vi "show_tag_status.vi"(11 "file path (dialog if empty)":path=path "c:/RFID/status.csv") -> (2 "Output":T2, 3 "train_passes_text":string)   [LabVIEW 2015]
uses:
  <vilib>/Utility/file.llb/Read Delimited Spreadsheet (string).vi
panel:
  out "all rows":string[][](array[string])
  in  "Cluster":T1
  out "subarray":string[](array[string])
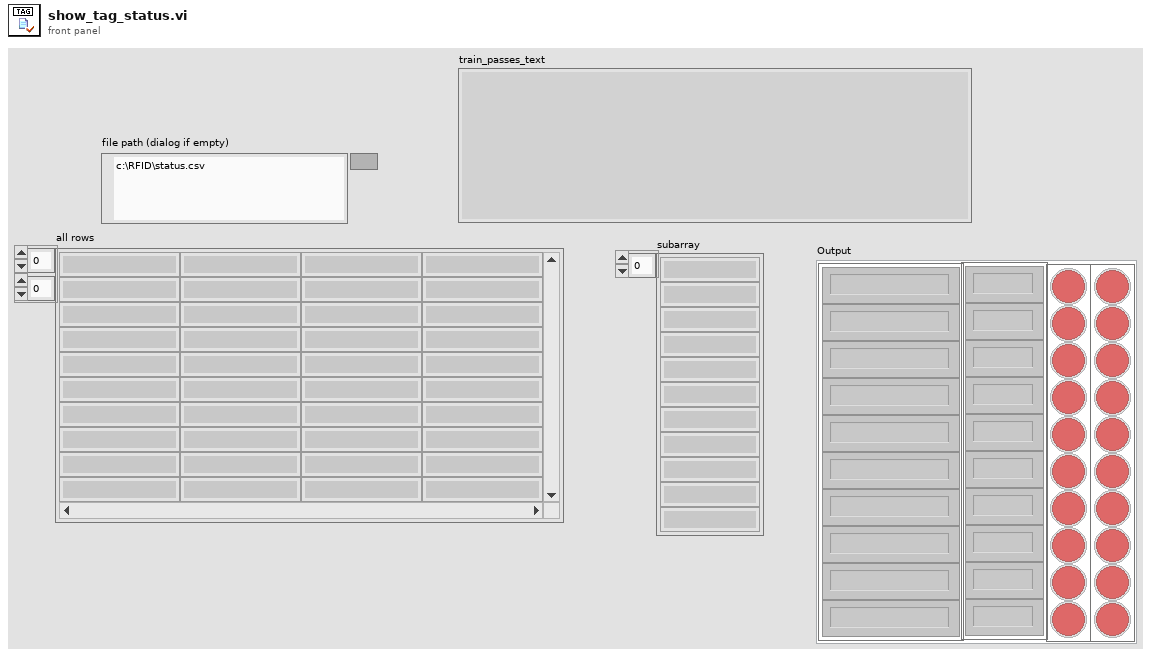
[diagram p1: front panel]
types:
  T1 = cluster{"Array 3":bool[], "Array 1":string[], "Array 2":string[], "Array 4":bool[]}
  T2 = cluster{"Array 3":bool[], "Array 4":string[], "Array 6":string[], "Array 5":bool[]}
  T3 = enum16{"open", "replace", "create", "open or create", "replace or create", "replace or create with confirmation"}
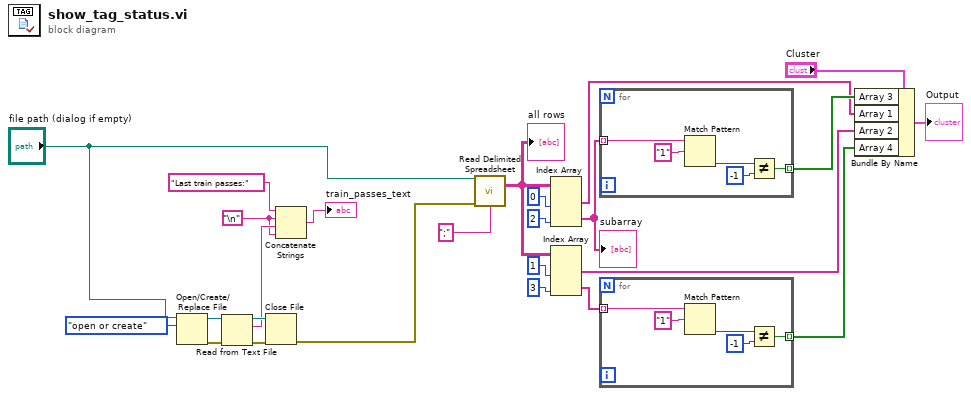
[diagram p0: block diagram]
diagram:
  w3 = "\n"
  n1 = Open/Create/Replace File(file path (use dialog)="file path (dialog if empty)", operation (0:open)=T3."open or create") -> (refnum out=w8:refnum<file>, error out=w10:errorcluster)  [unwired: 4 in, 1 out]
  n2 = Read from Text File(file (use dialog)=w8, error in=w10) -> (refnum out=w7:refnum<file>, text=w6:string, error out=w9:errorcluster)  [unwired: 2 in, 1 out]
  n3 = Close File(refnum=w7, error in=w9) -> (error out=w1:errorcluster)  [unwired: 1 out]
  n4 = Concatenate Strings("Last train passes:", w3, w6, w3) -> (→"train_passes_text":string)
  n5 = call-poly <vilib>:"Read Delimited Spreadsheet.vi"("file path (dialog if empty)"="file path (dialog if empty)", "error in (no error)"=w1, "delimiter (\\t)"=";" ("delimiter (\\t)")) -> ("all rows"=w12:string[][])  [unwired: 7 in, 5 out]
  "all rows" <- w12
  n6 = Index Array(array=w12, index (col) #1=0 ("index"), index (col) #2=2 ("index (col)")) -> (element #1=w19:string[], element #2=w21:string[])  [unwired: 2 in]
  "subarray" <- w21
  n7 = Index Array(array=w12, index (col) #1=1 ("index (col)"), index (col) #2=3 ("index (row)")) -> (element #1=w24:string[], element #2=w15:string[])  [unwired: 2 in]
  n8 = for {
    tunnel: w21 -> [w27] mode=indexing
    tunnel: [w26] -> w25 mode=indexing
    n9 = Match Pattern(string=w27, regular expression="1" ("element")) -> (offset past match=w28:i32)  [unwired: 1 in, 3 out]
    n10 = Not Equal?(x=w28, y=-1) -> (x != y?=w26:bool)
  }
  n11 = for {
    tunnel: w15 -> [w33] mode=indexing
    tunnel: [w31] -> w14 mode=indexing
    n12 = Match Pattern(string=w33, regular expression="1" ("element")) -> (offset past match=w32:i32)  [unwired: 1 in, 3 out]
    n13 = Not Equal?(x=w32, y=-1) -> (x != y?=w31:bool)
  }
  n14 = Bundle By Name(cluster="Cluster", "Array 3"=w25, "Array 1"=w19, "Array 2"=w24, "Array 4"=w14) -> (→"Output":T1)
